vi "Configure Fail Relay.vi"(0 "VISA resource name":refnum<visa-resource-name>, 1 "Communication Error (Off)":bool, 2 "Record Stop (Off)":bool, 3 "Alarm (Off)":bool, 5 "Fail Relay (0: Fail)":u16(ring) items=["Fail", "Status"], 7 "Memory/Media Status (Off)":bool, 9 "Measurement Error (Off)":bool, 11 "error in (no error)":errorcluster, 12 "Wireless Input Unit Error (Off)":bool) -> (4 "VISA resource name out":refnum<visa-resource-name>, 15 "error out":errorcluster)   [LabVIEW 2020, in "Yokogawa GX Series.lvlib"]
doc: "Sets the relay (DO channel) operation and the instrument status to output from the fail relay.\n\nCommands: SFailAct, SFailSts\n\nNote: This VI does nothing when the instrument is GM10."
uses:
  <instrlib>/Yokogawa GX Series/Yokogawa GX Series.lvlib
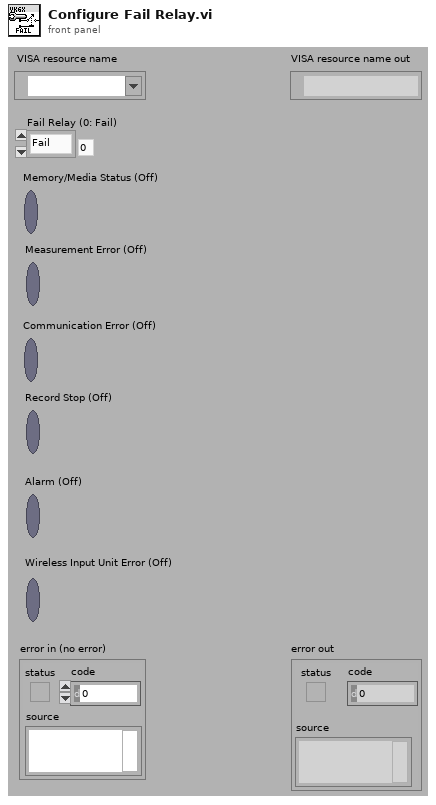
[diagram p1: front panel]
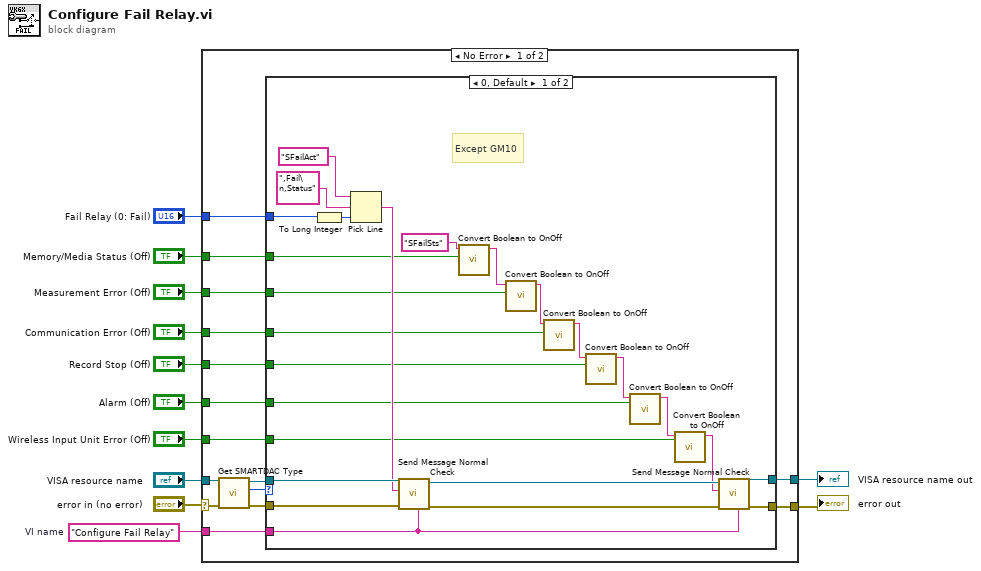
[diagram p0: block diagram]
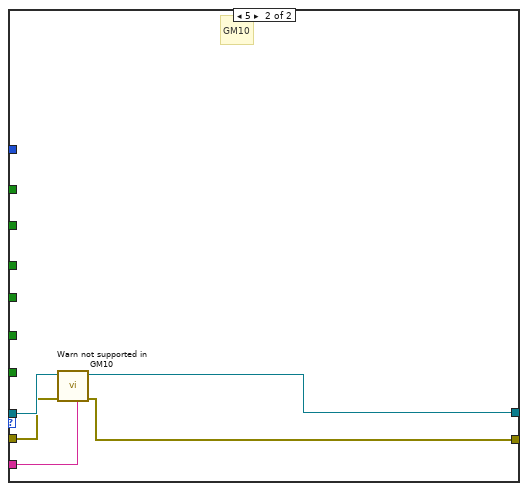
[diagram p2: hidden frame]
diagram:
  w8 = "Configure Fail Relay"  # VI name
  n1 = case shown="No Error" "error in (no error)" {
    selector: "error in (no error)" -> [w17 w58]
    tunnel: [w27 w59] -> w12
    tunnel: [w26 w58] -> w11
    tunnel: "VISA resource name" -> [w18 w59]
    tunnel: "Fail Relay (0: Fail)" -> [w25 _]
    tunnel: w8 -> [w24 _]
    tunnel: "Memory/Media Status (Off)" -> [w23 _]
    tunnel: "Measurement Error (Off)" -> [w22 _]
    tunnel: "Communication Error (Off)" -> [w21 _]
    tunnel: "Record Stop (Off)" -> [w20 _]
    tunnel: "Alarm (Off)" -> [w19 _]
    tunnel: "Wireless Input Unit Error (Off)" -> [w13 _]
    frame No Error {
      n2 = call <instrlib>:"Get SMARTDAC Type.vi"("error in (no error)"=w17, "VISA resource name"=w18) -> ("error out"=w15:errorcluster, "SMARTDAC+ Type"=w14:u16, "VISA resource name out"=w16:refnum<visa-resource-name>)  [unwired: 7 in]
      n3 = case shown="0, Default" w14 {
        tunnel: [w52 w55] -> w27
        tunnel: [w51 w54] -> w26
        tunnel: w16 -> [w50 w57]
        tunnel: w25 -> [w32 _]
        tunnel: w24 -> [w44 w53]
        tunnel: w23 -> [w42 _]
        tunnel: w22 -> [w40 _]
        tunnel: w21 -> [w31 _]
        tunnel: w20 -> [w37 _]
        tunnel: w19 -> [w35 _]
        tunnel: w15 -> [w34 w56]
        tunnel: w13 -> [w30 _]
        frame 0, Default {
          # "Except GM10"
          n4 = To Long Integer(number=w32) -> (32bit integer=w33:i32)
          n5 = Pick Line(string ("")="SFailAct", multi-line string=",Fail\n,Status", line index=w33) -> (output string=w45:string)
          n6 = call <instrlib>:"Send Message Normal Check.vi"("Source (\"\")"=w44, "error in (no error)"=w34, "Send Message (\"\")"=w45, "VISA resource name"=w50) -> ("error out"=w48:errorcluster, "VISA resource name out"=w49:refnum<visa-resource-name>)  [unwired: 2 in, 4 out]
          n7 = call <instrlib>:"Convert Boolean to OnOff.vi"("On/Off"=w42, "Initial String (\"\")"="SFailSts") -> ("Resulting String"=w41:string)  [unwired: 9 in]
          n8 = call <instrlib>:"Convert Boolean to OnOff.vi"("On/Off"=w40, "Initial String (\"\")"=w41) -> ("Resulting String"=w39:string)  [unwired: 9 in]
          n9 = call <instrlib>:"Convert Boolean to OnOff.vi"("On/Off"=w31, "Initial String (\"\")"=w39) -> ("Resulting String"=w38:string)  [unwired: 9 in]
          n10 = call <instrlib>:"Convert Boolean to OnOff.vi"("On/Off"=w37, "Initial String (\"\")"=w38) -> ("Resulting String"=w36:string)  [unwired: 9 in]
          n11 = call <instrlib>:"Convert Boolean to OnOff.vi"("On/Off"=w35, "Initial String (\"\")"=w36) -> ("Resulting String"=w29:string)  [unwired: 9 in]
          n12 = call <instrlib>:"Convert Boolean to OnOff.vi"("On/Off"=w30, "Initial String (\"\")"=w29) -> ("Resulting String"=w28:string)  [unwired: 9 in]
          n13 = call <instrlib>:"Send Message Normal Check.vi"("Source (\"\")"=w44, "error in (no error)"=w48, "Send Message (\"\")"=w28, "VISA resource name"=w49) -> ("error out"=w51:errorcluster, "VISA resource name out"=w52:refnum<visa-resource-name>)  [unwired: 2 in, 4 out]
        }
        frame 5 {
          # "GM10"
          n14 = call <instrlib>:"Warn not supported in GM10.vi"("Source (\"\")"=w53, "error in (no error)"=w56, "VISA resource name"=w57) -> ("error out"=w54:errorcluster, "VISA resource name out"=w55:refnum<visa-resource-name>)  [unwired: 7 in]
        }
      }
    }
    frame Error {
    }
  }
  "error out" <- w11
  "VISA resource name out" <- w12
